vi "rvc Plot 2D Transform.vi"   [LabVIEW 2017]
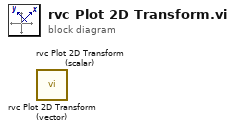
[diagram p0: block diagram]
diagram:
  n1 = call "rvc Plot 2D Transform (vector).vi"() -> ()  [unwired: 10 in, 2 out]
  n2 = call "rvc Plot 2D Transform (scalar).vi"() -> ()  [unwired: 10 in, 2 out]
